vi "dfd_PR Cosine-Modulated Initialize Param.vi"(7 "M":i32=4, 10 "roll off":dbl=0.99, 11 "order":i32=39) -> (3 "Initial phi":dbl[](array[numeric]), 5 "param":cluster{"M":i32, "Us":dbl[][], "roll off":dbl})   [LabVIEW 2017, in "NI_DigFilter_FilterBank.lvlib"]
uses:
  <vilib>/addons/Digital Filter Design/NI_DigFilter_FilterBank.lvlib
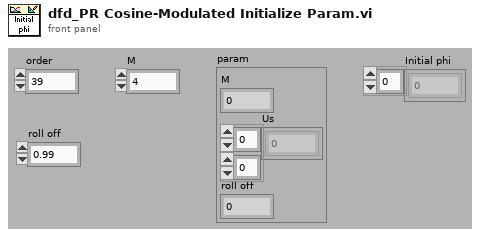
[diagram p1: front panel]
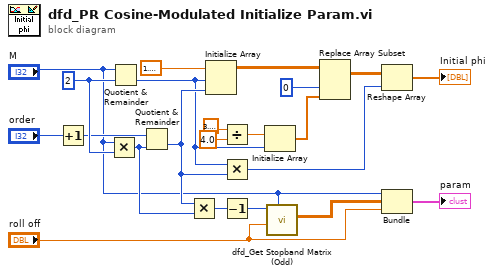
[diagram p0: block diagram]
diagram:
  w20 = 2 ("y")
  n1 = Increment(x="order") -> (x+1=w19:i32)
  n2 = Multiply(x="M", y=w20) -> (x*y=w5:i32)
  n3 = Quotient & Remainder(x="M", y=w20) -> (floor(x/y)=w7:i32)  [unwired: 1 out]
  n4 = Quotient & Remainder(x=w19, y=w5) -> (floor(x/y)=w8:i32)  [unwired: 1 out]
  n5 = Multiply(x=w8, y=w5) -> (x*y=w4:i32)
  n6 = Initialize Array(1.5707963267948966, w7, w8) -> (w18:dbl[][])
  n7 = Divide(x=3.141592653589793, y=4.0) -> (x/y=w14:dbl)
  n8 = Multiply(x=w7, y=w8) -> (x*y=w9:i32)
  n9 = Decrement(x=w4) -> (x-1=w12:i32)
  n10 = Initialize Array(w14, w7) -> (w13:dbl[])
  n11 = call <vilib>:"dfd_Get Stopband Matrix (Odd).vi"("number of bands"="M", "roll off"="roll off", "order"=w12) -> ("Us"=w11:dbl[][])  [unwired: 8 in]
  n12 = Replace Array Subset(array=w18, new element=w13, index (col)=0 ("disabled index (col)")) -> (w10:dbl[][])  [unwired: 1 in]
  n13 = Reshape Array(w10, w9) -> (→"Initial phi":dbl[])
  n14 = Bundle("M"="M", "Us"=w11, "roll off"="roll off") -> (→"param":cluster{"M":i32, "Us":dbl[][], "roll off":dbl})  [unwired: 1 in]
